vi "grab image.vi"() -> ()   [LabVIEW 2018]
uses:
  <vilib>/userdefined/High Color/IMAQdx.ctl
  <vilib>/vision/driver/NI_Vision_Acquisition_Software.lvlib
panel:
  in  "Session In":T1
  out "Buffer Number Out":u32
  in  "정지 버튼":bool
  out "Image":T2(plugin-control)
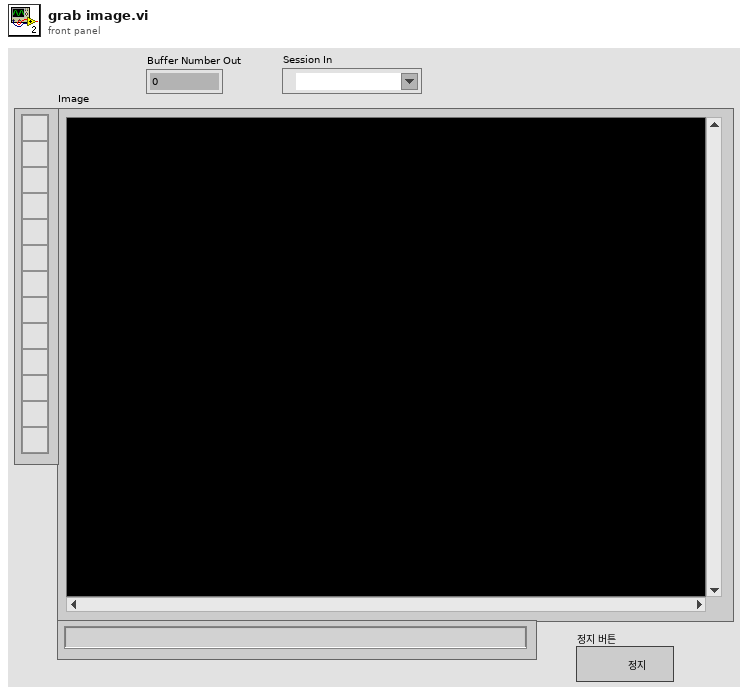
[diagram p1: front panel]
types:
  T1 = typedef "IMAQdx.ctl" = refnum<k21>
  T2 = typedef "IMAQ Image.ctl" = refnum<image>
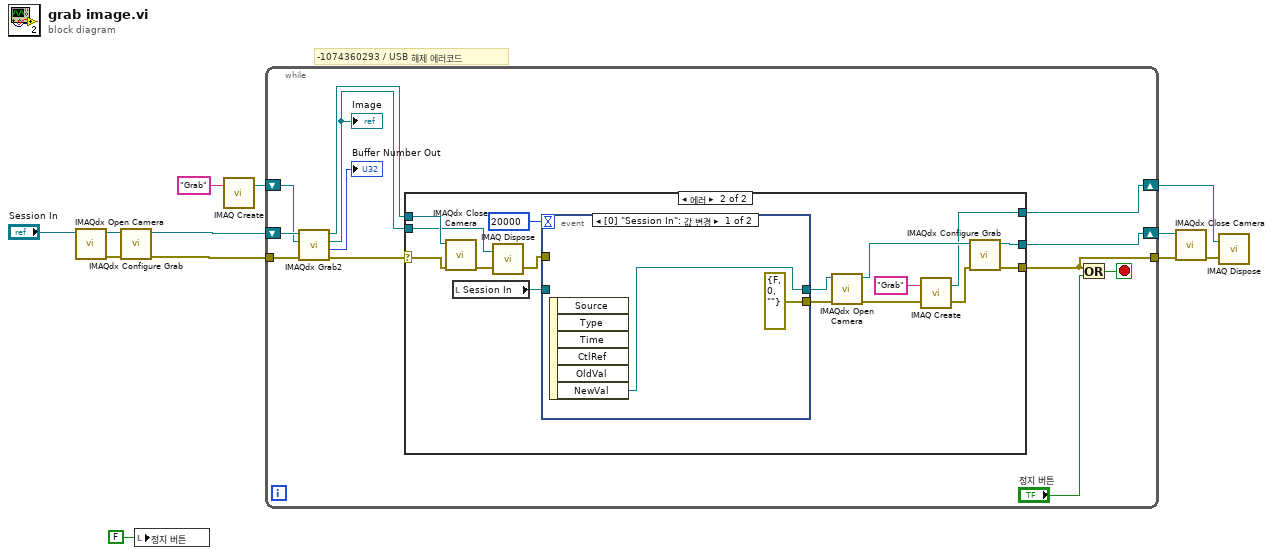
[diagram p0: block diagram]
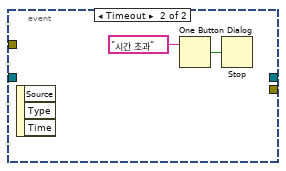
[diagram p3: hidden frame]
diagram:
  # "-1074360293 / USB 해제 에러코드"
  n1 = call <vilib>:"IMAQdx Open Camera.vi"("Session In"="Session In") -> ("error out"=w10:errorcluster, "Session Out"=w11:T1)  [unwired: 9 in]
  n2 = call <vilib>:"IMAQdx Configure Grab.vi"("error in"=w10, "Session In"=w11) -> ("error out"=w8:errorcluster, "Session Out"=w9:T1)  [unwired: 8 in]
  n3 = local write "정지 버튼"(FALSE ("정지 버튼")) -> ()
  n4 = call "IMAQ Create"("Image Name"="Grab") -> ("New Image"=w5:T2)  [unwired: 4 in, 1 out]
  n5 = while {
    tunnel: w8 -> [w23]
    tunnel: [w13] -> w7
    shift-right: [w17] -> w2
    shift-left: w9 -> [w24]
    shift-right: [w15] -> w1
    shift-left: w5 -> [w19]
    stop <- w21 stop-if-true
    n6 = call <vilib>:"IMAQdx Grab2.vi"("error in"=w23, "Image In"=w19, "Session In"=w24) -> ("error out"=w14:errorcluster, "Buffer Number Out"=→"Buffer Number Out":u32, "Image Out"=w16:T2, "Session Out"=w18:T1)  [unwired: 5 in]
    "Image" <- w16
    n7 = case shown="에러" w14 {
      selector: w14 -> [w27 w42]
      tunnel: [w27 w35] -> w13
      tunnel: w18 -> [w26 w41]
      tunnel: [w26 w34] -> w17
      tunnel: w16 -> [w25 w40]
      tunnel: [w25 w33] -> w15
      frame No Error {
      }
      frame Error {
        n8 = call <vilib>:"IMAQdx Close Camera.vi"("error in"=w42, "Session In"=w41) -> ("error out"=w43:errorcluster)  [unwired: 9 in]
        n9 = local read "Session In"() -> (w32:T1)
        n10 = call "IMAQ Dispose"("Image"=w40, "error in (no error)"=w43) -> ("error out"=w29:errorcluster)  [unwired: 4 in]
        n11 = event shown="[0] \"Session In\": 값 변경" {
          selector: _ -> [_ _]
          dyn-events: _ -> [_ _]
          timeout: 20000 -> [_ _]
          tunnel: w32 -> [_ _]
          tunnel: [w45 _] -> w31
          tunnel: w29 -> [_ _]
          tunnel: [errorcluster {"status"=FALSE, "code"=0, "source"=""} ("error out") _] -> w28
          event Value Change {
            n12 = event-data() -> ("NewVal"=w45:T1)  [unwired: 1 in, 5 out]
          }
          event Timeout {
            n13 = event-data() -> ()  [unwired: 1 in, 3 out]
            n14 = One Button Dialog(message="시간 초과" ("메시지")) -> (true=w46:bool)  [unwired: 1 in]
            n15 = Stop(stop? (T)=w46) -> ()
          }
        }
        n16 = call <vilib>:"IMAQdx Open Camera.vi"("error in"=w28, "Session In"=w31) -> ("error out"=w38:errorcluster, "Session Out"=w37:T1)  [unwired: 8 in]
        n17 = call "IMAQ Create"("Image Name"="Grab", "error in (no error)"=w38) -> ("New Image"=w33:T2, "error out"=w36:errorcluster)  [unwired: 3 in]
        n18 = call <vilib>:"IMAQdx Configure Grab.vi"("error in"=w36, "Session In"=w37) -> ("error out"=w35:errorcluster, "Session Out"=w34:T1)  [unwired: 8 in]
      }
    }
    n19 = Or(x=w13, y="정지 버튼") -> (x .or. y?=w21:bool)
  }
  n20 = call <vilib>:"IMAQdx Close Camera.vi"("error in"=w7, "Session In"=w2) -> ("error out"=w6:errorcluster)  [unwired: 9 in]
  n21 = call "IMAQ Dispose"("Image"=w1, "error in (no error)"=w6) -> ()  [unwired: 4 in, 1 out]
